vi "valves_write.vi"(8 "error in (no error)":errorcluster, 9 "Valves":bool[](array[boolean]), 10 "Channel":string="A", 11 "Port ref out":refnum<k24>) -> (0 "error out":errorcluster, 3 "Port ref in":refnum<k24>)   [LabVIEW 2018]
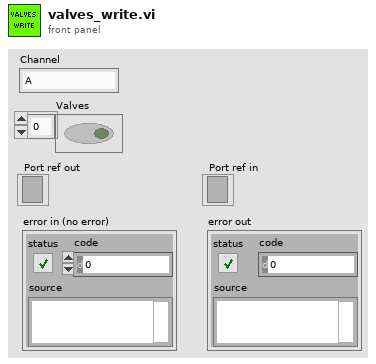
[diagram p1: front panel]
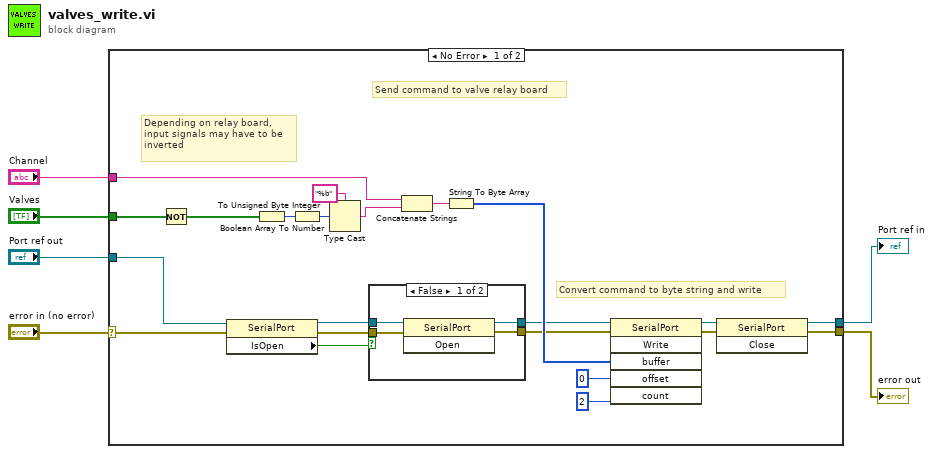
[diagram p0: block diagram]
diagram:
  n1 = case shown="No Error" "error in (no error)" {
    selector: "error in (no error)" -> [w9 w36]
    tunnel: [w26 w35] -> w6
    tunnel: [w25 w36] -> w5
    tunnel: "Port ref out" -> [w24 w35]
    tunnel: "Valves" -> [w8 _]
    tunnel: "Channel" -> [w11 _]
    frame No Error {
      # "Depending on relay board,\ninput signals may have to be\ninverted"
      # "Convert command to byte string and write"
      # "Send command to valve relay board"
      n2 = Not(x=w8) -> (.not. x?=w7:bool[])
      n3 = property class="SerialPort"(reference=w24, error in=w9) -> (reference out=w23:refnum<k24>, error out=w22:errorcluster, "IsOpen"=w28:bool)
      n4 = Boolean Array To Number(Boolean array=w7) -> (number=w12:u32)
      n5 = To Unsigned Byte Integer(number=w12) -> (unsigned 8bit integer=w13:u8)
      n6 = Type Cast(type="%b", x=w13) -> (*(type *) &x=w15:string)
      n7 = case shown="False" w28 {
        tunnel: [w31 w34] -> w20
        tunnel: [w30 w33] -> w21
        tunnel: w23 -> [w32 w34]
        tunnel: w22 -> [w29 w33]
        frame False {
          n8 = invoke class="SerialPort" method="Open"(reference=w32, error in=w29) -> (reference out=w31:refnum<k24>, error out=w30:errorcluster)  [unwired: 1 in, 1 out]
        }
        frame True {
        }
      }
      n9 = Concatenate Strings(w11, w15) -> (w10:string)
      n10 = String To Byte Array(string=w10) -> (unsigned byte array=w27:u8[])
      n11 = invoke class="SerialPort" method="Write"(reference=w20, error in=w21, "buffer"=w27, "offset"=0, "count"=2) -> (reference out=w18:refnum<k24>, error out=w19:errorcluster)  [unwired: 1 in, 4 out]
      n12 = invoke class="SerialPort" method="Close"(reference=w18, error in=w19) -> (reference out=w26:refnum<k24>, error out=w25:errorcluster)  [unwired: 1 in, 1 out]
    }
    frame Error {
    }
  }
  "error out" <- w5
  "Port ref in" <- w6
